vi "Create.vi"(10 "API ID":string) -> (3 "ApiIdentity out":refnum<class "ApiIdentity.lvclass">)   [LabVIEW 2020, in "Volatus.lvlib" / "ApiIdentity.lvclass"]
uses:
  ApiIdentity.lvclass
  ApiIdentity.lvclass/ApiIdentity.ctl
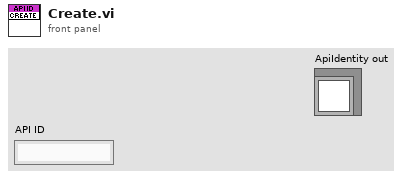
[diagram p1: front panel]
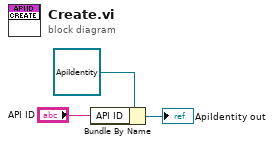
[diagram p0: block diagram]
diagram:
  n1 = Bundle By Name(cluster=refnum<class "ApiIdentity.lvclass"> refnum ("ApiIdentity in"), "API ID"="API ID") -> (→"ApiIdentity out":refnum<class "ApiIdentity.lvclass">)
